vi "To Distance.vi"(2 "Tolerance":dbl=2.5 format="%#_13g", 3 "Destination Dist (in)":dbl, 4 "Min. Power":dbl, 5 "Reset":bool) -> (0 "Reached Distance":bool, 1 "Base Speed":dbl)   [LabVIEW 2014]
panel:
  in  "Inches to Max Power":dbl=120.0 format="%#_13g"
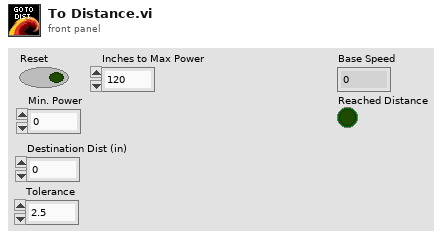
[diagram p1: front panel]
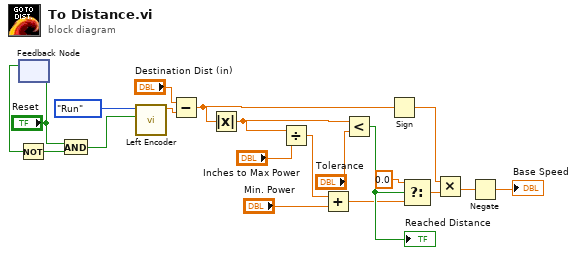
[diagram p0: block diagram]
diagram:
  n1 = feedback-in #1("Reset") -> ()
  n2 = feedback #1() -> (w5:bool)  [unwired: 1 in]
  n3 = Not(x=w5) -> (.not. x?=w6:bool)
  n4 = And(x="Reset", y=w6) -> (x .and. y?=w4:bool)
  n5 = call "Left Encoder.vi"("Reset"=w4, "Enum"=enum16{"Start", "Run", "End"}."Run") -> ("Distance (in)"=w7:dbl)  [unwired: 8 in, 1 out]
  n6 = Subtract(x="Destination Dist (in)", y=w7) -> (x-y=w9:dbl)
  n7 = Absolute Value(x=w9) -> (abs(x)=w17:dbl)
  n8 = Divide(x=w17, y="Inches to Max Power") -> (x/y=w15:dbl)
  n9 = Add(x=w15, y="Min. Power") -> (x+y=w13:dbl)
  n10 = Less?(x=w17, y="Tolerance") -> (x < y?=w19:bool)
  "Reached Distance" <- w19
  n11 = Sign(1:w9) -> (0:w11:dbl)
  n12 = Select(t=0.0, s=w19, f=w13) -> (s? t:f=w12:dbl)
  n13 = Multiply(x=w11, y=w12) -> (x*y=w2:dbl)
  n14 = Negate(x=w2) -> (-x=→"Base Speed":dbl)
